vi "rvc Generate Multi-segment trajectory.vi"(6 "initial coordinate axis":dbl[](array[numeric]), 7 "Duration for  segments?":bool, 9 "time steps":dbl, 10 "velocity limits":dbl[](array[numeric]), 11 "segments":dbl[][](array[numeric])) -> ()   [LabVIEW 2013]
uses:
  <vilib>/robotics/Kinematics/NI_Kinematics.lvlib
  <vilib>/robotics/Kinematics/Generate Joint Trajectory (Int).vi
panel:
  out "tseg":dbl
  out "s? t:f":dbl
  in  "acceleration limits":dbl[](array[numeric])
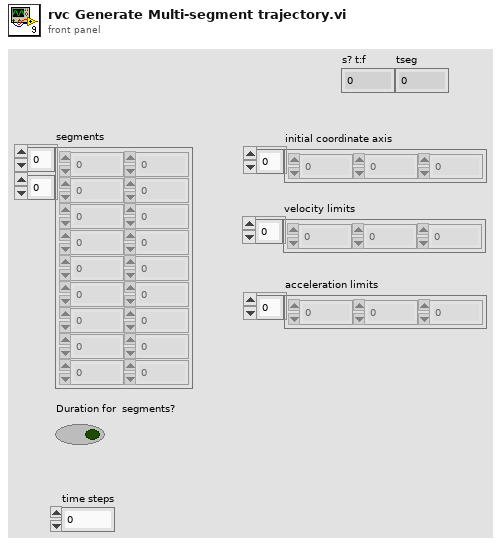
[diagram p1: front panel]
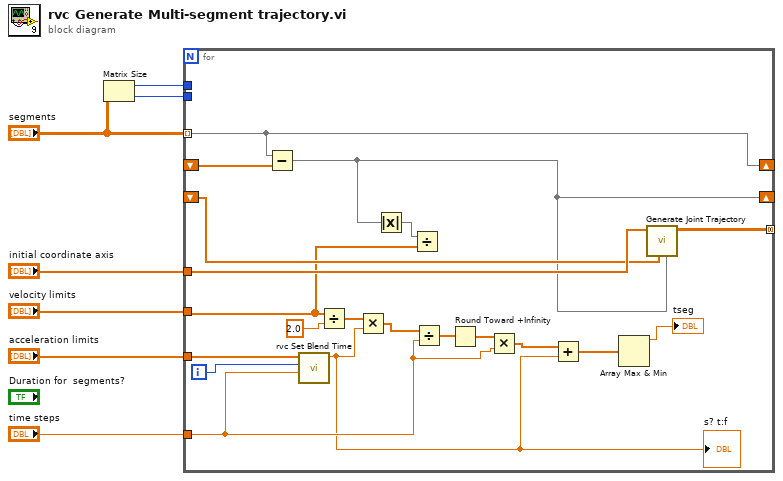
[diagram p0: block diagram]
diagram:
  n1 = Matrix Size(0:"segments") -> (1:w1:i32, 2:w3:i32)
  n2 = for {
    tunnel: "segments" -> [w24] mode=indexing
    tunnel: "initial coordinate axis" -> [w23]
    tunnel: "velocity limits" -> [w16]
    tunnel: "acceleration limits" -> [w27]
    tunnel: w1 -> [_]
    tunnel: w3 -> [_]
    tunnel: "time steps" -> [w12]
    shift-right: [w24] -> _
    shift-left: _ -> [w25]
    shift-right: [w18] -> _
    shift-left: _ -> [w22]
    tunnel: [w21] -> _ mode=concatenating
    i -> [w26]
    n3 = Subtract(x=w24, y=w25) -> (x-y=w18:dbl[])
    n4 = call "rvc Set Blend Time.vi"("time steps"=w12, "seg"=w26, "acceleration limits"=w27) -> ("taccx"=w10:dbl)  [unwired: 6 in, 2 out]
    "s? t:f" <- w10
    n5 = Divide(x=w16, y=2.0 ("taccx")) -> (x/y=w20:dbl[])
    n6 = Multiply(x=w20, y=w10) -> (x*y=w15:dbl[])
    n7 = Absolute Value(x=w18) -> (abs(x)=w17:dbl[])
    n8 = Divide(x=w17, y=w16) -> ()  [unwired: 1 out]
    n9 = Divide(x=w15, y=w12) -> (x/y=w14:dbl[])
    n10 = Round Toward +Infinity(x=w14) -> (ceil(x): smallest int >= x=w13:dbl[])
    n11 = Multiply(x=w13, y=w12) -> (x*y=w11:dbl[])
    n12 = Add(x=w11, y=w10) -> (x+y=w9:dbl[])
    n13 = Array Max & Min(array=w9) -> (max value=→"tseg":dbl)  [unwired: 3 out]
    n14 = call-poly <vilib>:"Generate Joint Trajectory.vi"("end joint velocities"=w18, "start joint velocities"=w22, "start joint positions"=w23) -> ("joint position trajectory"=w21:dbl[][])  [unwired: 5 in, 3 out]
  }
